vi "My Global Var.vi"() -> ()   [LabVIEW 2017]
panel:
  in  "Setup Description":string="0 - Channel Setup\n1 - PID Setup\n2 - Filter Setup\n3 - ~Reserved Old CAN MSG\n4 - ~Reserved Old CAN 1\n5 - ~Reserved Old CAN 2\n6 - Digital Inputs Setup\n7 - Digital Outputs Setup\n8 - Logging 1 Setup\n9 - Logging 2 Setup\n10 - Logging 3 Setup\n11 - Setpoint Setup\n12 - Test Series Setup\n13 - Graph Setup\n14 - System Configure\n15 - Header\n16 - Profile Manager\n17 - Post-Mortem Logging\n18 - High-Speed Data\n19 - Statistic Channel Setup\n20 - Ramp Channel Setup\n21 - ETAS INCA Channel Setup\n22 - ETC ECCS Transducer Setup\n23 - ETC ECCS Test Setup\n24 - AVL AK Smoke Meter Setup\n25 - Triggers Setup\n26 - Alarm Limits Setup\n27 - YKWT1 Measurement\n28 - YKWT1 Instrument\n29 - Auto File Settings\n30 - Playback File Setting\n31 - UUT Constants\n32 - UPS Setup\n33 - Differential Channel Setup\n34 - Integral Channel Setup\n35 - Signal Channel Setup\n36 - Calibration Setup\n37 - BNC Setup\n38 - ASAP3 Setup\n39 - Chassis Force Calculations\n40 - Chassis Teststand Losses\n41 - Chassis Vehicle Losses\n42 - Formula Channels\n43 - ASAP3 Map Coords Setup\n44 - Digital Controls Setup\n45 - Push Buttons Setup\n46 - Sliders Setup\n47 - ~Reserved~\n48 - Email Setup\n49 - Timer Setup\n50 - Unit Conversion Setup\n51 - Visible Channels\n52 - Main Display Setup\n53 - Message Display Setup\n54 - Input Display Setup\n55 - Unico Parameter Downloads\n56 - Flow Meter Setup\n57 - Channel Zero Offset\n58 - YKWT2 Measurement\n59 - YKWT2 Instrument\n60 - ~Reserved Old CAN 3\n61 - CAS Setup\n62 - Accumulation Channel Setup\n63 - Valvetrain Dynamics Setup\n64 - CCP Setup\n65 - System Log Setup\n66 - Throttle Controller\n67 - RE Shifter\n68 - Main Display\n69 - ~Reserved~\n70 - FlexRay\n71 - YKWT3 Measurement\n72 - YKWT3 Instrument\n73 - CAN XNET API"
  in  "Setup Pattern":string=".chn\n.pid\n.fil\n.cnm\n.can\n.can\n.dis\n.dos\n.lgg\n.lgg\n.lgg\n.spt\n.tss\n.grp\n.cfs\n.hdr\n.pmgr\n.lgg\n.hsd\n.mth\n.rsf\n.inc\n.ecx\n.ect\n.avl\n.trg\n.lts\n.msr\n.wt3\n.afn\n.pla\n.uut\n.ups\n.dff\n.int\n.sig\n.cal\n.bnc\n.as3\n.cls\n.tls\n.vls\n.frm\n.am3\n.dcs\n.pbs\n.scs\n.afi\n.eml\n.tmr\n.ucv\n.vchn\n.mds\n.mdp\n.inp\n.uni\n.fms\n.chzo\n.msr\n.wt3\n.can\n.cas\n.cml\n.vtd\n.ccp\n.syl\n.tcrl\n.csv\n.mdsp\n.exa\n.flex\n.msr\n.wt3\n.cxt"
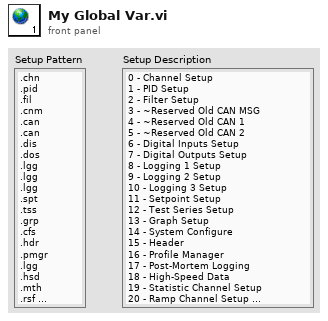
[diagram p1: front panel]
diagram:
